vi "genRandStreamStim.vi"(8 "error in (no error)":errorcluster, 10 "Queue length trigger":i32=1, 11 "Stim in":refnum<class "Stim.lvclass">) -> (0 "error out":errorcluster, 2 "# elements in queue":i32, 3 "Stim out":refnum<class "Stim.lvclass">)   [LabVIEW 2014, in "Stim.lvclass"]
uses:
  Stim.lvclass
  Stim.lvclass/Stim.ctl
panel:
  in  "Stim Queue":T1
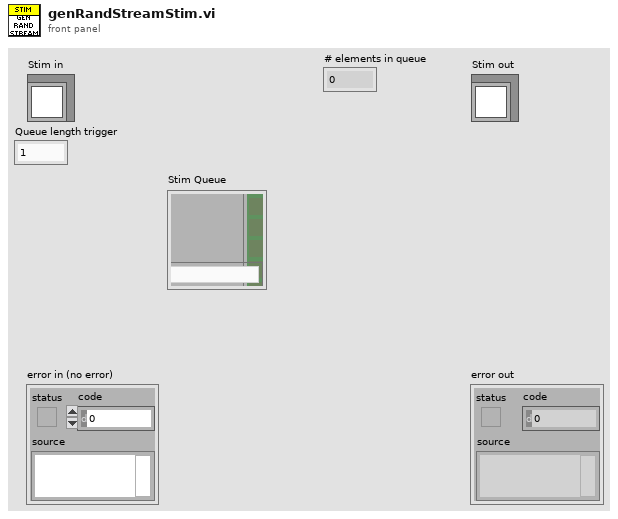
[diagram p1: front panel]
types:
  T1 = cluster{"Stimulus channels":bool[], "Stimulus":string}
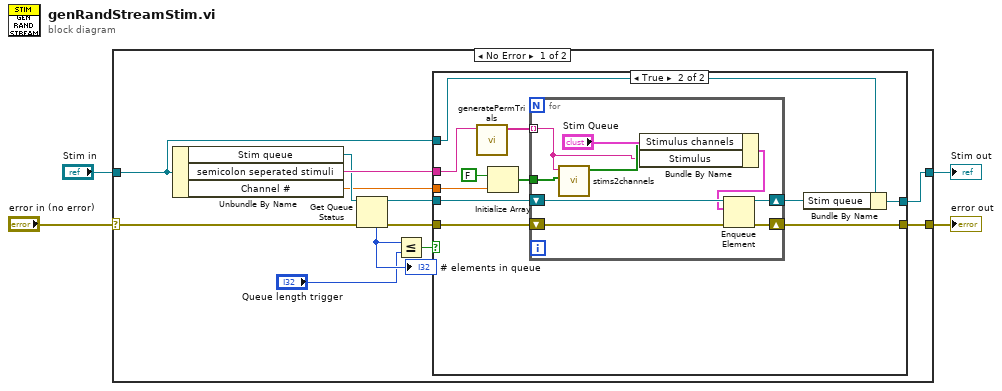
[diagram p0: block diagram]
diagram:
  n1 = case shown="No Error" "error in (no error)" {
    selector: "error in (no error)" -> [w10 w40]
    tunnel: [w16 w40] -> w3
    tunnel: [w14 w39] -> w2
    tunnel: "Stim in" -> [w15 w39]
    frame No Error {
      n2 = Unbundle By Name(w15) -> ("Stim queue"=w12:refnum<queue>, "semicolon seperated stimuli"=w13:string, "Channel #"=w5:dbl)
      n3 = Get Queue Status(queue=w12, error in (no error)=w10) -> (queue out=w11:refnum<queue>, error out=w9:errorcluster, # elements in queue=w8:i32)  [unwired: 1 in, 5 out]
      "# elements in queue" <- w8
      n4 = Less Or Equal?(x=w8, y="Queue length trigger") -> (x <= y?=w6:bool)
      n5 = case shown="True" w6 {
        tunnel: w9 -> [w17 w28]
        tunnel: [w17 w27] -> w16
        tunnel: w15 -> [w18 w26]
        tunnel: [w18 w25] -> w14
        tunnel: w13 -> [_ w23]
        tunnel: w11 -> [_ w22]
        tunnel: w5 -> [_ w19]
        frame False {
        }
        frame True {
          n6 = call "generatePermTrials.vi"("semicolon seperated stimuli"=w23) -> ("perfmutated trials"=w29:string[])  [unwired: 9 in, 1 out]
          n7 = Initialize Array(FALSE, w19) -> (w20:bool[])
          n8 = for {
            shift-right: [w37] -> w27
            shift-left: w28 -> [w38]
            shift-right: [w35] -> w24
            shift-left: w22 -> [w36]
            tunnel: w29 -> [w31] mode=indexing
            tunnel: w20 -> [w34]
            n9 = call "stims2channels.vi"("Stimulus channel array"=w34, "Stimuli"=w31) -> ("Stimulus channels"=w32:bool[])  [unwired: 9 in]
            n10 = Bundle By Name(cluster="Stim Queue", "Stimulus channels"=w32, "Stimulus"=w31) -> (w30:T1)
            n11 = Enqueue Element(queue=w36, element=w30, error in (no error)=w38) -> (queue out=w35:refnum<queue>, error out=w37:errorcluster)  [unwired: 1 in, 1 out]
          }
          n12 = Bundle By Name(cluster=w26, "Stim queue"=w24) -> (w25:refnum<class "Stim.lvclass">)
        }
      }
    }
    frame Error {
    }
  }
  "error out" <- w3
  "Stim out" <- w2
